vi "holoCodeOrHoloDir.vi"(7 "Radio bottons":i32, 8 "HoloList Reff":refnum<vi>, 10 "HoloHelp Reff":refnum<vi>, 11 "HoloCode Reff":refnum<vi>) -> ()   [LabVIEW 2023]
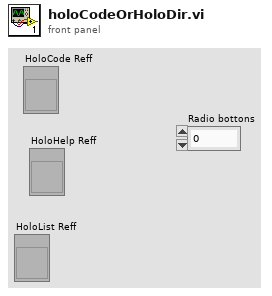
[diagram p1: front panel]
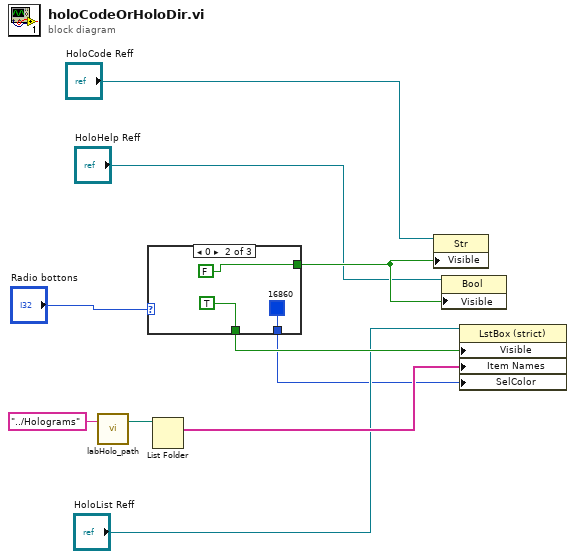
[diagram p0: block diagram]
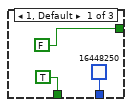
[diagram p2: hidden frame]
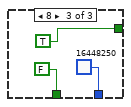
[diagram p3: hidden frame]
diagram:
  n1 = call "labHolo_path.vi"("sub folder or file (str)"="../Holograms") -> ("labHolo path"=w9:path)  [unwired: 1 in, 1 out]
  n2 = case shown="0" "Radio bottons" {
    tunnel: [FALSE FALSE TRUE] -> w7
    tunnel: [TRUE TRUE FALSE] -> w6
    tunnel: [u32 16448250 ("Selection Color") u32 16860 ("Selection Color") u32 16448250 ("Selection Color")] -> w1
    frame 1, Default {
    }
    frame 0 {
    }
    frame 8 {
    }
  }
  n3 = List Folder(path=w9) -> (filenames=w5:string[])  [unwired: 3 in, 3 out]
  n4 = property on="Property Node" class="Str"(reference="HoloCode Reff", "Visible"=w7) -> ()  [unwired: 1 in, 2 out]
  n5 = property on="Property Node" class="Bool"(reference="HoloHelp Reff", "Visible"=w7) -> ()  [unwired: 1 in, 2 out]
  n6 = property on="Property Node" class="LstBox (strict)"(reference="HoloList Reff", "Visible"=w6, "Item Names"=w5, "SelColor"=w1) -> ()  [unwired: 1 in, 2 out]
